vi "数字至2位字符串转换.vi"(11 "数值":i32) -> (3 "数据字符串":string)   [LabVIEW 2016]
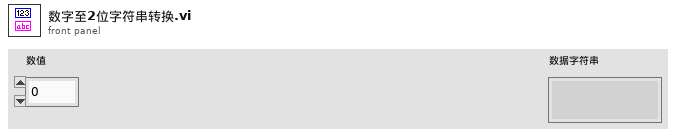
[diagram p1: front panel]
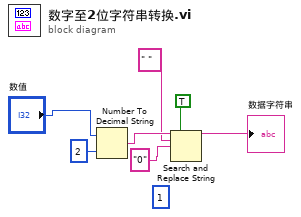
[diagram p0: block diagram]
diagram:
  (unwired) 1 ("长度（子字符串长度）")
  n1 = Number To Decimal String(number="数值", width (-)=i16 2 ("宽度(-)")) -> (decimal integer string=w5:string)
  n2 = Search and Replace String(replace all?=TRUE ("替换全部？(F)"), input string=w5, search string=" " ("搜索字符串"), replace string="0" ("子字符串(\"\")")) -> (result string=→"数据字符串":string)  [unwired: 4 in, 3 out]
